vi "complete_with_zero.vi"(1 "#Chars":i32=6, 2 "Number":i32) -> (5 "StringOut":string)   [LabVIEW 2018]
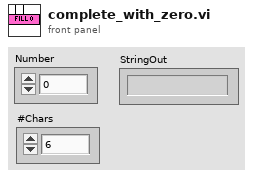
[diagram p1: front panel]
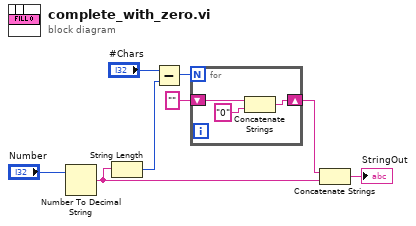
[diagram p0: block diagram]
diagram:
  n1 = Number To Decimal String(number="Number") -> (decimal integer string=w3:string)  [unwired: 1 in]
  n2 = String Length(string=w3) -> (length=w7:i32)
  n3 = Subtract(x="#Chars", y=w7) -> (x-y=w5:i32)
  n4 = for {
    N: w5 -> [_]
    shift-right: [w10] -> w4
    shift-left: "" -> [w9]
    n5 = Concatenate Strings(w9, "0") -> (w10:string)
  }
  n6 = Concatenate Strings(w4, w3) -> (→"StringOut":string)
